vi "Configure Channel (mA Delta).vi"(0 "VISA resource name":refnum<visa-resource-name>, 1 "Reference Channel (0001)":string="0001", 5 "Channel (0001)":string="0001", 7 "Enable Channel (True)":bool=TRUE, 9 "Span":T1={"mA Range (0 : 0-20mA)"=0, "Enable Span (False)"=FALSE, "Lower Span (0.000)"=0.0, "Upper Span (20.000)"=20.0, "Bias (0)"=0.0} {"mA Range (0 : 0-20mA)" items=["0-20mA"]; "Bias (0)" format="%_6g"; "Upper Span (20.000)" step=0.001 format="%.3g"; "Lower Span (0.000)" step=0.001 format="%.3g"}, 11 "error in (no error)":errorcluster) -> (4 "VISA resource name out":refnum<visa-resource-name>, 6 "Channel":string, 15 "error out":errorcluster)   [LabVIEW 2020, in "Yokogawa GX Series.lvlib"]
doc: "Sets the input range as voltage.\n\nCommand: SRangeAI"
uses:
  <instrlib>/Yokogawa GX Series/Yokogawa GX Series.lvlib
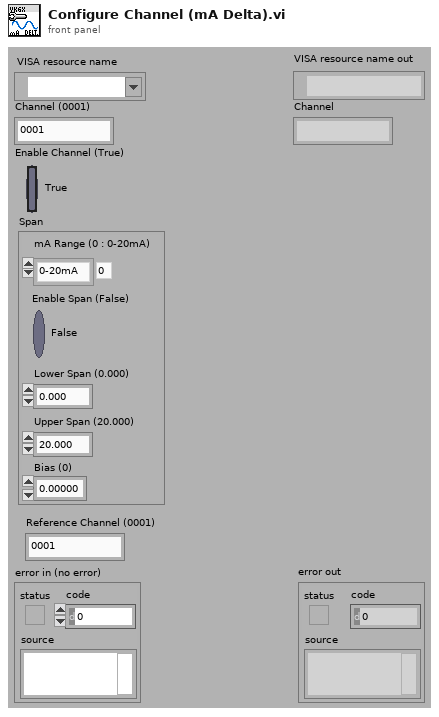
[diagram p1: front panel]
types:
  T1 = cluster{"mA Range (0 : 0-20mA)":i32, "Enable Span (False)":bool, "Lower Span (0.000)":dbl, "Upper Span (20.000)":dbl, "Bias (0)":dbl}
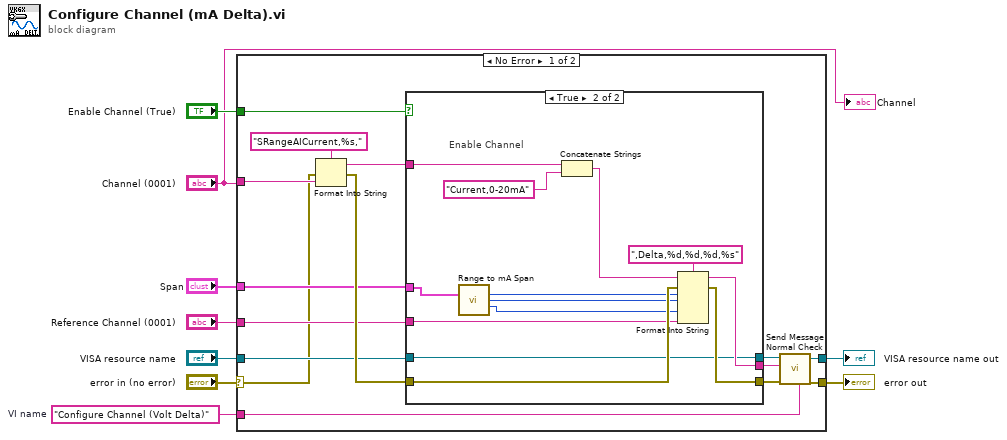
[diagram p0: block diagram]
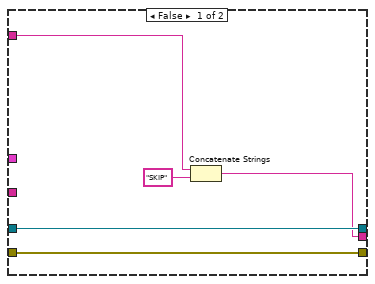
[diagram p2: hidden frame]
diagram:
  w5 = "Configure Channel (Volt Delta)"  # VI name
  n1 = case shown="No Error" "error in (no error)" {
    selector: "error in (no error)" -> [w10 w43]
    tunnel: "Enable Channel (True)" -> [w21 _]
    tunnel: "VISA resource name" -> [w20 w44]
    tunnel: [w18 w44] -> w7
    tunnel: [w17 w43] -> w6
    tunnel: w5 -> [w14 _]
    tunnel: "Span" -> [w13 _]
    tunnel: "Reference Channel (0001)" -> [w12 _]
    tunnel: "Channel (0001)" -> [w11 _]
    frame No Error {
      n2 = Format Into String(format string="SRangeAICurrent,%s,", error in=w10, w11) -> (resulting string=w22:string, error out=w23:errorcluster)  [unwired: 1 in]
      n3 = case shown="True" w21 {
        tunnel: w23 -> [w28 w38]
        tunnel: w12 -> [_ w36]
        tunnel: [w28 w40] -> w19
        tunnel: w22 -> [w29 w41]
        tunnel: w20 -> [w26 w37]
        tunnel: [w26 w37] -> w15
        tunnel: [w25 w39] -> w16
        tunnel: w13 -> [_ w34]
        frame False {
          n4 = Concatenate Strings(w29, "SKIP") -> (w25:string)
        }
        frame True {
          # "Enable Channel"
          n5 = call <instrlib>:"Range to mA Span.vi"("Span"=w34) -> ("Lower Span"=w33:i32, "Upper Span"=w32:i32, "Bias"=w31:i32)  [unwired: 12 in]
          n6 = Concatenate Strings(w41, "Current,0-20mA") -> (w30:string)
          n7 = Format Into String(format string=",Delta,%d,%d,%d,%s", initial string=w30, error in=w38, w33, w32, w31, w36) -> (resulting string=w39:string, error out=w40:errorcluster)
        }
      }
      n8 = call <instrlib>:"Send Message Normal Check.vi"("Source (\"\")"=w14, "error in (no error)"=w19, "Send Message (\"\")"=w16, "VISA resource name"=w15) -> ("error out"=w17:errorcluster, "VISA resource name out"=w18:refnum<visa-resource-name>)  [unwired: 2 in, 4 out]
    }
    frame Error {
    }
  }
  "error out" <- w6
  "VISA resource name out" <- w7
  "Channel" <- "Channel (0001)"
